vi "gen_laservoltage_sequence_samples.vi"(0 "V min":dbl, 5 "V max":dbl, 7 "# V steps":dbl, 11 "# Samples per voltage point":i32) -> (6 "Voltage sequence":dbl[](array[numeric]), 10 "Total # data points":i32)   [LabVIEW 2012]
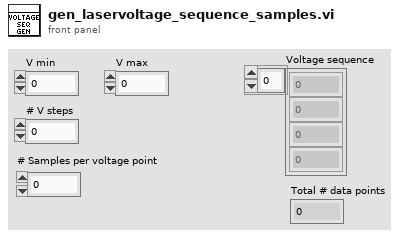
[diagram p1: front panel]
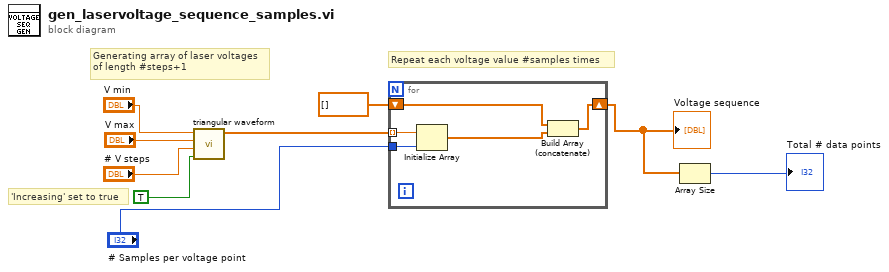
[diagram p0: block diagram]
diagram:
  # "Repeat each voltage value #samples times"
  # "'Increasing' set to true"
  # "Generating array of laser voltages\nof length #steps+1"
  n1 = call "triangular waveform.vi"("Increasing?"=TRUE, "# of steps"="# V steps", "max"="V max", "min"="V min") -> ("data"=w5:dbl[])  [unwired: 7 in]
  n2 = for {
    tunnel: w5 -> [w14] mode=indexing
    tunnel: "# Samples per voltage point" -> [w13]
    shift-right: [w10] -> w2
    shift-left: dbl[] [] ("appended array") -> [w12]
    n3 = Initialize Array(w14, w13) -> (w11:dbl[])
    n4 = Build Array (concatenate)(w12, w11) -> (w10:dbl[])
  }
  "Voltage sequence" <- w2
  n5 = Array Size(array=w2) -> (size(s)=→"Total # data points":i32)
